vi "MotionProfiles_NewPoints.vi"(8 "error in (no error)":errorcluster, 10 "CSV File Path":path=path "/home/lvuser/mp.csv", 11 "MotionProfiles in":refnum<class "MotionProfiles.lvclass">) -> (0 "error out":errorcluster, 3 "MotionProfiles out":refnum<class "MotionProfiles.lvclass">)   [LabVIEW 2017, in "MotionProfiles.lvclass"]
uses:
  MotionProfiles.lvclass
  MotionProfile_TrajectoryPoint.ctl
  MotionProfile_InternalStateEnum.ctl
  MotionProfile_TalonSetValueEnum.ctl
  MotionProfiles.lvclass/MotionProfiles.ctl
  <vilib>/Utility/file.llb/Read Delimited Spreadsheet (DBL).vi
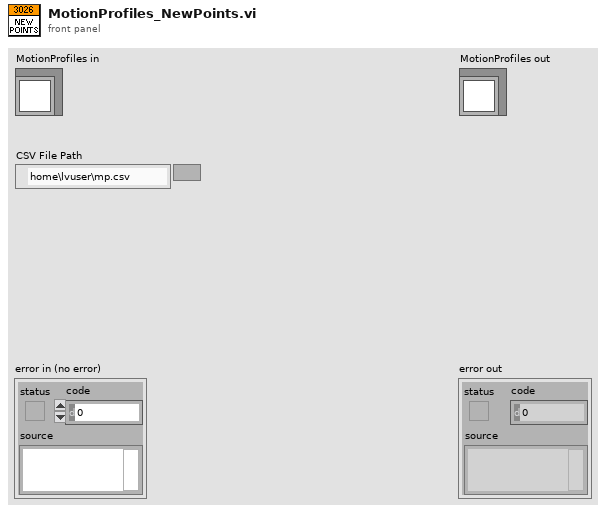
[diagram p1: front panel]
types:
  T1 = typedef "MotionProfiles.lvclass/MotionProfile_TalonSetValueEnum.ctl" = enum16{"Disable", "Enable", "Hold"}
  T2 = typedef "MotionProfiles.lvclass/MotionProfile_InternalStateEnum.ctl" = enum16{"Nothing", "Send Points to Talon", "Run Profile"}
  T3 = typedef "MotionProfiles.lvclass/MotionProfile_TrajectoryPoint.ctl" = cluster{"Duration (ms)":u8, "Velocity (u/100ms)":dbl, "Position (units)":dbl, "Profile Slot Select":u8, "Is Last":bool, "Velocity Only":bool, "Zero Position":bool, "Compress Code":u8, "Same Velocity":i32, "Delta Position":i32, "Count":u8, "Invert Motors?":bool}
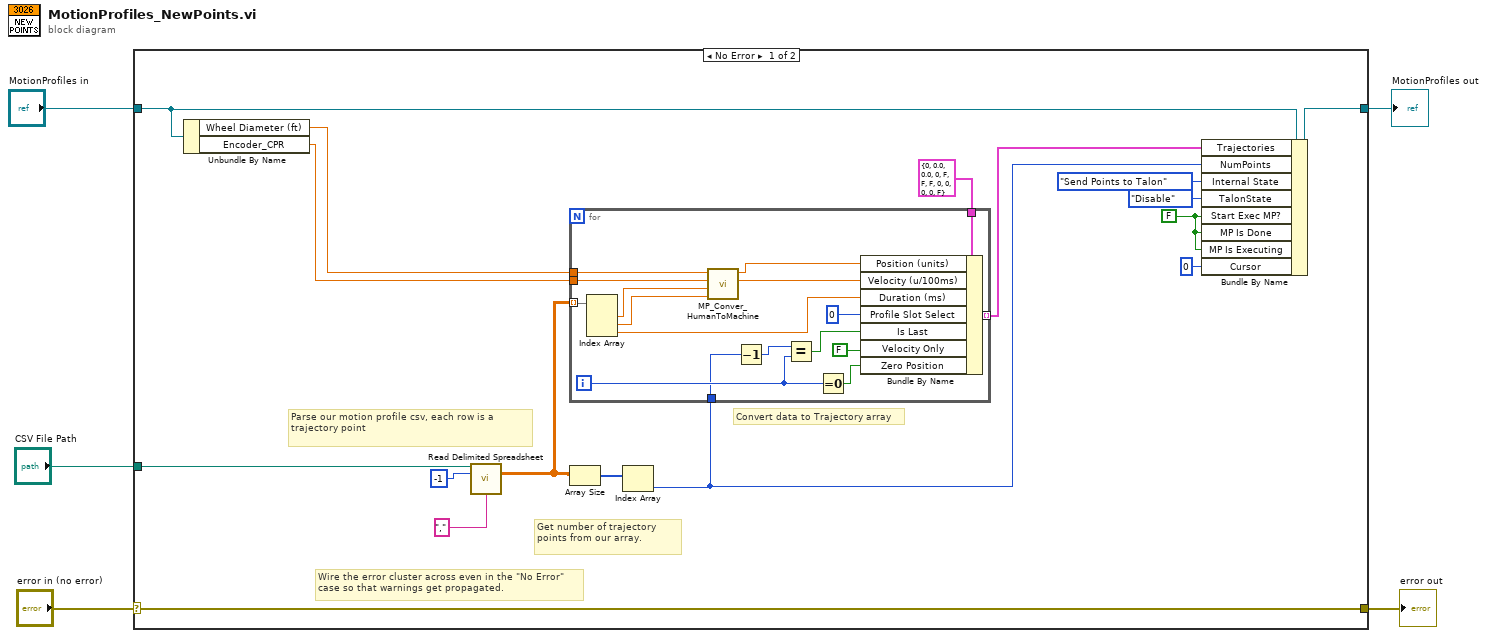
[diagram p0: block diagram]
diagram:
  n1 = case shown="No Error" "error in (no error)" {
    selector: "error in (no error)" -> [w22 w41]
    tunnel: [w22 w41] -> w4
    tunnel: [w21 w40] -> w2
    tunnel: "MotionProfiles in" -> [w20 w40]
    tunnel: "CSV File Path" -> [w13 _]
    frame No Error {
      w7 = FALSE ("Start Exec MP?")
      # "Convert data to Trajectory array"
      # "Get number of trajectory points from our array."
      # "Parse our motion profile csv, each row is a trajectory point"
      # "Wire the error cluster across even in the \"No Error\"\ncase so that warnings get propagated."
      n2 = Unbundle By Name(w20) -> ("Wheel Diameter (ft)"=w15:dbl, "Encoder_CPR"=w14:dbl)
      n3 = call-poly <vilib>:"Read Delimited Spreadsheet.vi"("file path (dialog if empty)"=w13, "number of rows (all:-1)"=-1, "delimiter (\\t)"="," ("delimiter (\\t)")) -> ("all rows"=w17:dbl[][])  [unwired: 7 in, 5 out]
      n4 = Array Size(array=w17) -> (size(s)=w16:i32[])
      n5 = Index Array(array=w16) -> (element=w10:i32)  [unwired: 1 in]
      n6 = for {
        tunnel: [w37] -> w11 mode=indexing
        tunnel: w17 -> [w35] mode=indexing
        tunnel: w10 -> [w30]
        tunnel: w15 -> [w27]
        tunnel: w14 -> [w26]
        tunnel: T3 {"Duration (ms)"=0, "Velocity (u/100ms)"=0.0, "Position (units)"=0.0, "Profile Slot Select"=0, "Is Last"=FALSE, "Velocity Only"=FALSE, "Zero Position"=FALSE, "Compress Code"=0, "Same Velocity"=0, "Delta Position"=0, "Count"=0, "Invert Motors?"=FALSE} ("Motion Profile Trajectory Point") -> [w23]
        i -> [w32]
        n7 = Index Array(array=w35) -> (element #1=w25:dbl, element #2=w24:dbl, element #3=w34:dbl)  [unwired: 3 in]
        n8 = call "MP_Conver_HumanToMachine.vi"("Vel_In (ft/s)"=w24, "Pos_In (ft)"=w25, "CPR"=w26, "Diameter (ft)"=w27) -> ("Vel_Out (u/100ms)"=w28:dbl, "Pos_Out (u)"=w29:dbl)  [unwired: 4 in]
        n9 = Decrement(x=w30) -> (x-1=w31:i32)
        n10 = Equal?(x=w31, y=w32) -> (x = y?=w33:bool)
        n11 = Equal To 0?(x=w32) -> (x = 0?=w38:bool)
        n12 = Bundle By Name(cluster=w23, "Position (units)"=w29, "Velocity (u/100ms)"=w28, "Duration (ms)"=w34, "Profile Slot Select"=u8 0, "Is Last"=w33, "Velocity Only"=FALSE, "Zero Position"=w38) -> (w37:T3)
      }
      n13 = Bundle By Name(cluster=w20, "Trajectories"=w11, "NumPoints"=w10, "Internal State"=MotionProfile_InternalStateEnum."Send Points to Talon", "TalonState"=MotionProfile_TalonSetValueEnum."Disable", "Start Exec MP?"=w7, "MP Is Done"=w7, "MP Is Executing"=w7, "Cursor"=u32 0) -> (w21:refnum<class "MotionProfiles.lvclass">)
    }
    frame Error {
    }
  }
  "error out" <- w4
  "MotionProfiles out" <- w2
